vi "GUI_Mlink_Heater.vi"() -> ()   [LabVIEW 2013]
uses:
  Shared/GUI_Template/GUI_master/tcp_new_data_event.ctl
  Shared/GUI_Template/GUI_master/tcp new data cluster.ctl
  <vilib>/Utility/config.llb/Read Key (String).vi
  <vilib>/Utility/config.llb/NI_LVConfig.lvlib
panel:
  in  "Tab Control":enum32{"Plot history", "Configuration", "Debug"}(tab)
  out "Ch1 2":cluster{dbl[], dbl[]}[](graph)
  out "Ch1":cluster{dbl[], dbl[]}[](graph)
  in  "Calibration file path":string="user data\\PL_Energy_meter_callibration.txt"
  in  "Target propagation (%)":dbl=73.68421 format="%_6g"
  in  "Attenuator 2.1 transmittance (%)":dbl format="%_6g"
  in  "Attenuator 2.2 transmittance (%)":dbl=10.1068 format="%_6g"
  in  "Attenuator 1 transmittance (%)":dbl=1.83867 format="%_6g"
  in  "mirror offset (mJ)":dbl
  in  "mirror transmittance (%)":dbl=5.0 format="%_6g"
  out "GUIdevice 1":string="LB-PL-EnergyMeter"
  in  "Select device":string(combo)="LB-PL-EnergyMeter"
  in  "datastream::1":enum16{"off", "on"}(ring)
  in  "polarity::1":enum16{"Positive", "Negative"}(ring) caption="Trigger Polarity"
  out "validdata::1":enum16{"yes", "no"}(ring)
  out "error":errorcluster
  in  "Attenuator 2":enum16{"Out", "In (Att. 2.1)", "In (Att. 2.2)"}(ring)
  in  "Attenuator 1":enum16{"In", "Out"}(ring)=enum."Out"
  in  "Position powermeter":enum16{"In beamline", "Behind mirror"}(ring)=enum."Behind mirror"
  in  "Scale":T1(ring)
  in  "trigger::1":enum16{"Internal", "External"}(ring) caption="Trigger"
  in  "autorange::1":enum16{"off", "on"}(ring) caption="AutoRange"
  out "Target energy (J)":dbl=25.5 min=0.0 max=300000000.0 format="%#_6p"
  out "Full beam energy (J)":dbl=25.5 min=0.0 max=300000000.0 format="%#_6p"
  in  "stop":bool
  in  "data::1":dbl=25.5 caption="Raw energy (J)" min=0.0 max=300000000.0 format="%#_6p"
  in  "Clear 2":bool
  out "tcp data event 2":T2
  in  "insert tag":bool=TRUE
  # "HPD Energy Meter"
  # "Settings"
  # "Aditional settings"
  # "Setup parameters"
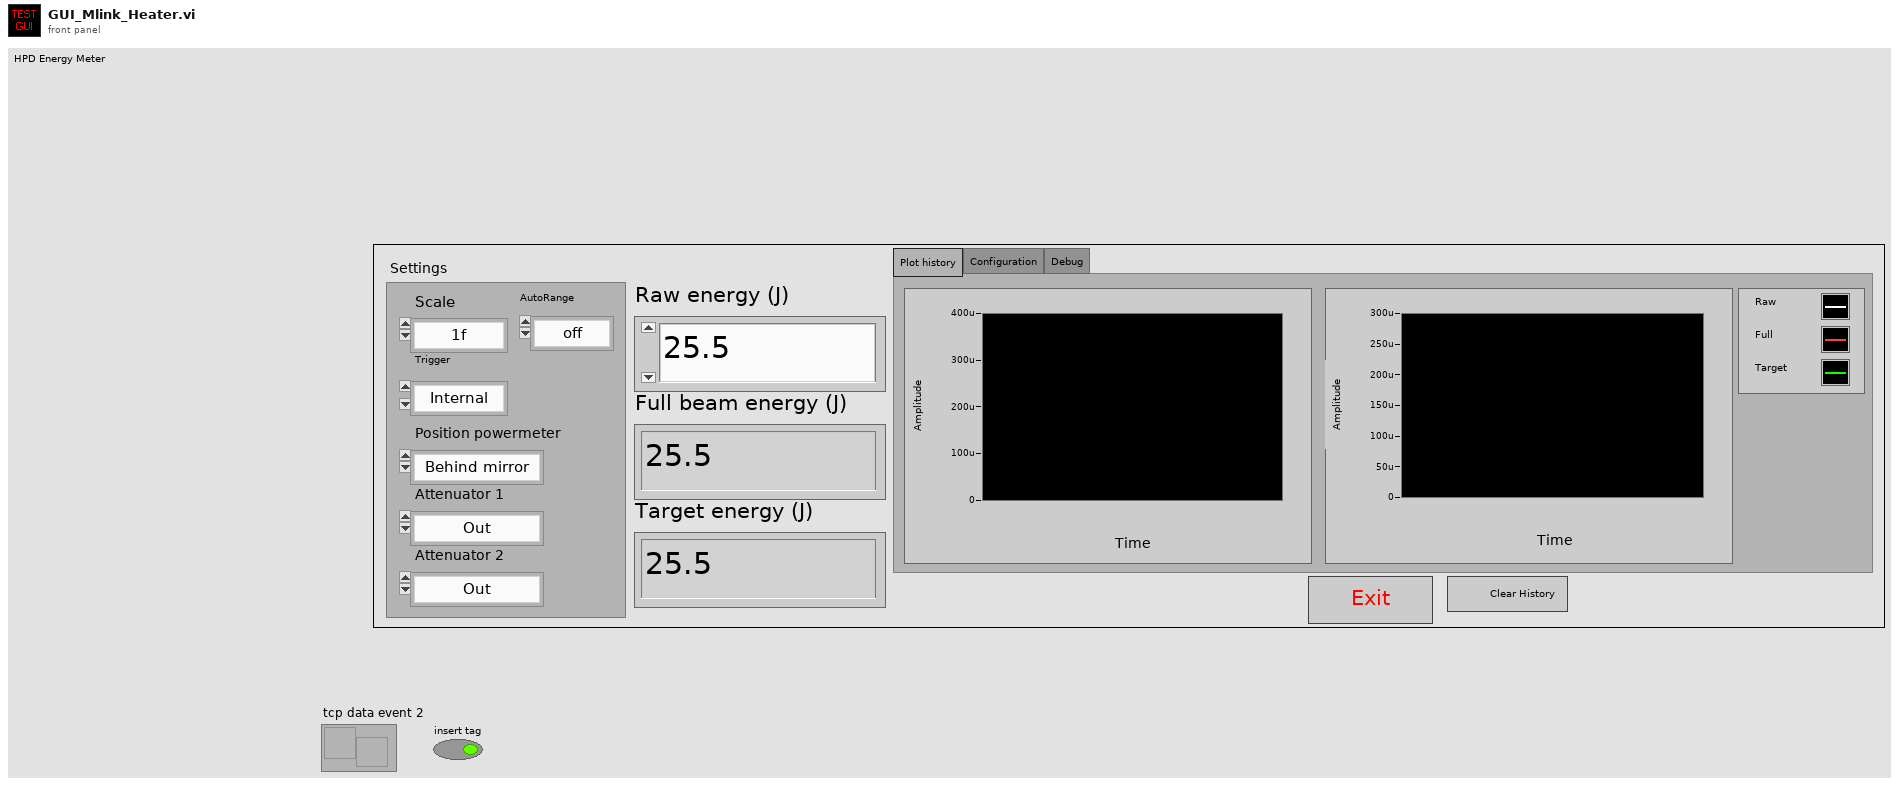
[diagram p1: front panel]
types:
  T1 = enum16{"1f", "3f", "10f", "30f", "100f", "300f", "1p", "3p", "10p", "30p", "100p", "300p", "1n", "3n", "10n", "30n", "100n", "300n", "1u", "3u", "10u", "30u", "100u", "300u", "1m", "3m", "10m", "30m", "100m", "300m", "1", "3", "10", "30", "100", "300", "1K", "3K", "10K", "30K", "100K", "300K", "1M", "3M", "10M", "30M", "100M", "300M"}
  T2 = typedef "tcp_new_data_event.ctl" = refnum<user-event>
  T3 = enum32{"invalid app kind", "Development System", "Run Time System", "Student Edition", "Embedded LabVIEW", "Evaluation", "Custom"}
  T4 = typedef "tcp new data cluster.ctl" = cluster{"EventEnum":enum16{"new data", "connection status update"}, "Device name":string}
  T5 = enum32{"Invalid", "Standard", "Closed", "Hidden", "Minimized", "Maximized"}
  T6 = cluster{"Core":cluster{"Current VI Reference":refnum<vi>, "Close Panel on Exit?":bool}, "Your Boolean data":bool, "Your string data":string, "SuperGUI":cluster{"STOP queue":refnum<queue>, "SuperGUI ref":refnum<vi>, "event reg":refnum<event-registration>}, "Timer":u32, "Raw energy":dbl, "Full energy":dbl, "Target energy":dbl, "Display Error Popup":bool}
  T7 = cluster{"STOP queue":refnum<queue>, "SuperGUI ref":refnum<vi>, "event reg":refnum<event-registration>}
  T8 = cluster{"Current VI Reference":refnum<vi>, "Close Panel on Exit?":bool}
  T9 = typedef "NI_LVConfig.lvlib/Config Data RefNum.ctl" = refnum<k1>
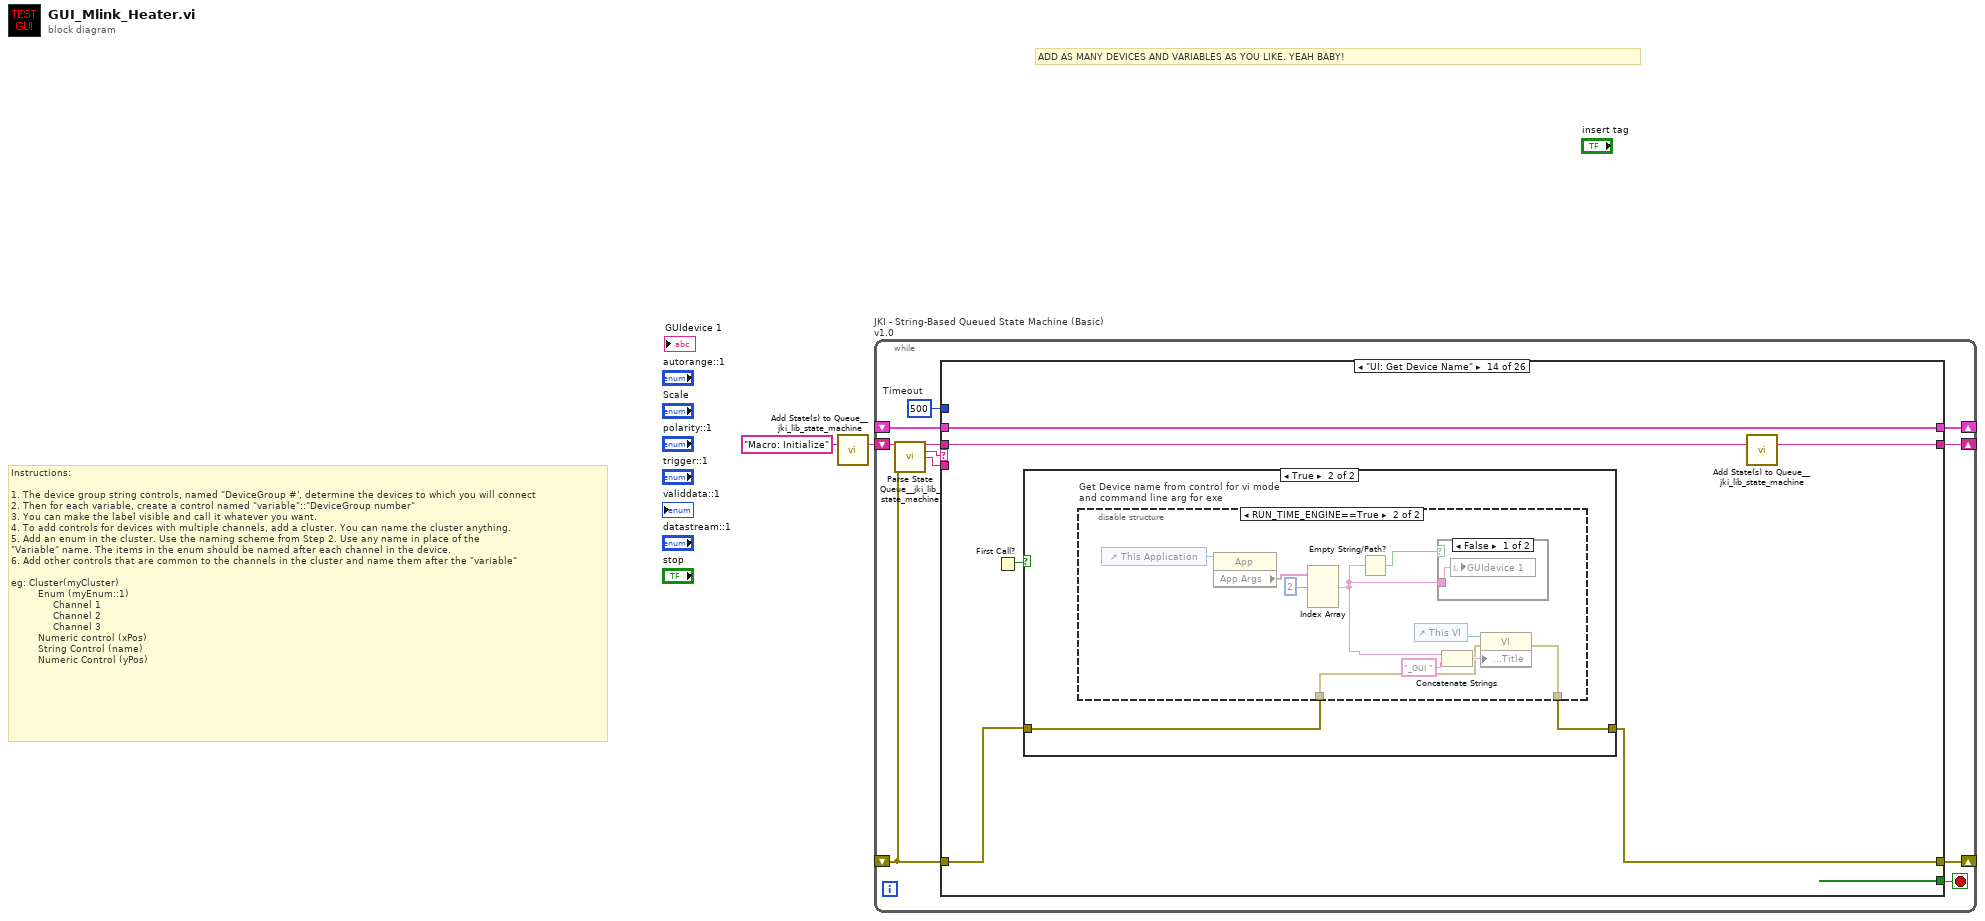
[diagram p0: block diagram]
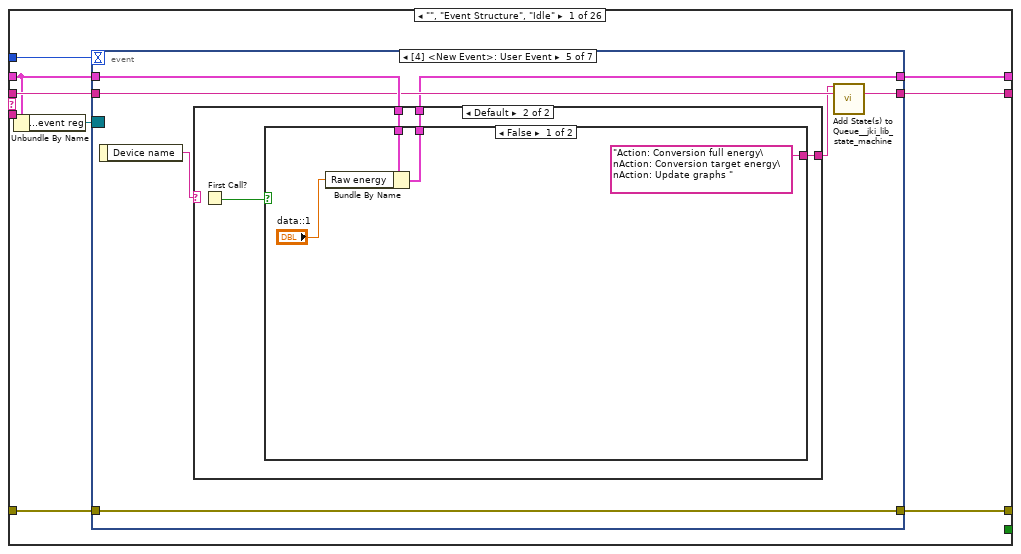
[diagram p2: hidden frame]
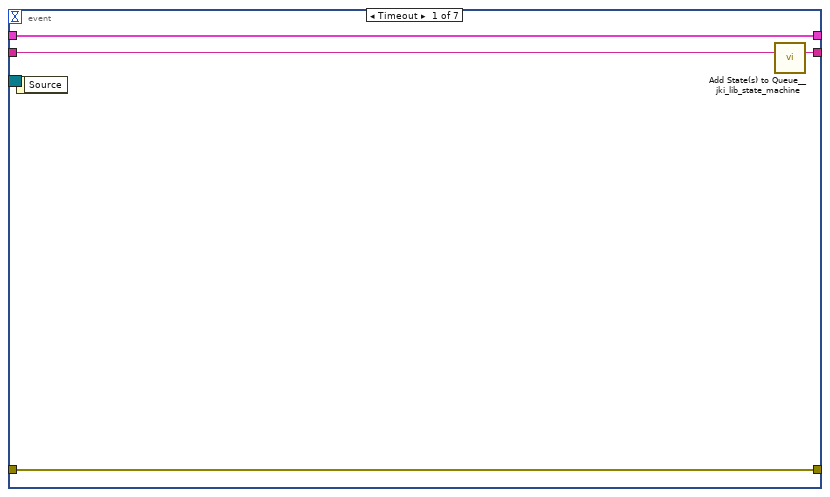
[diagram p3: hidden frame]
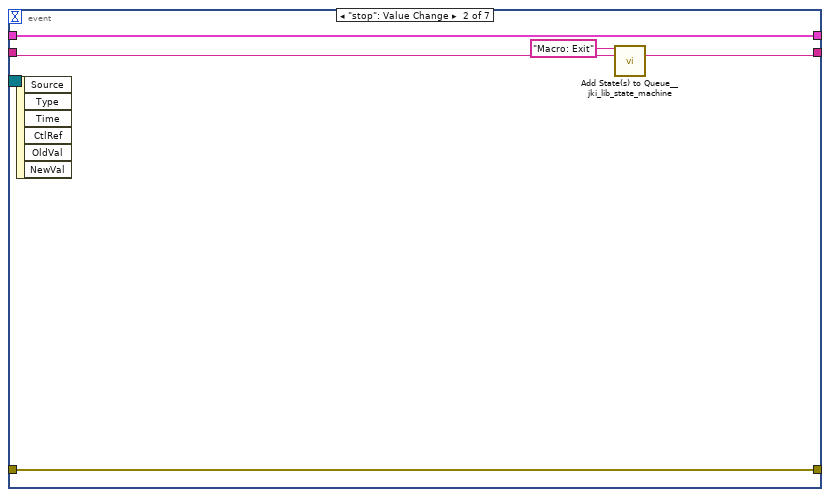
[diagram p4: hidden frame]
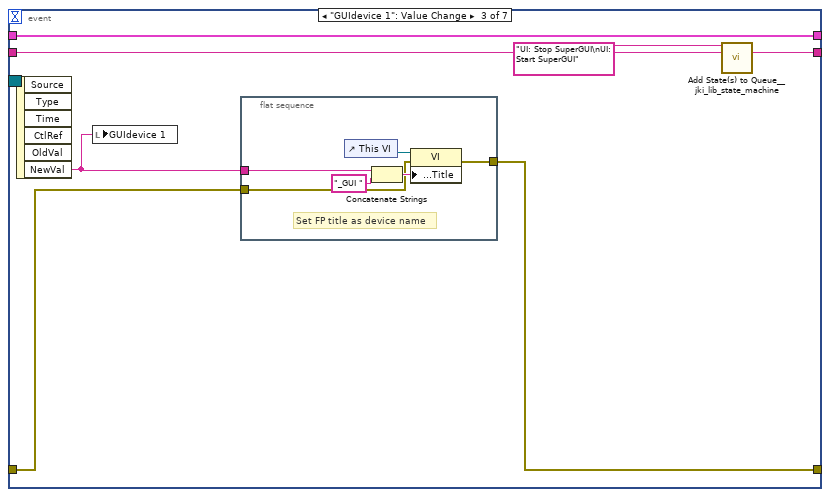
[diagram p5: hidden frame]
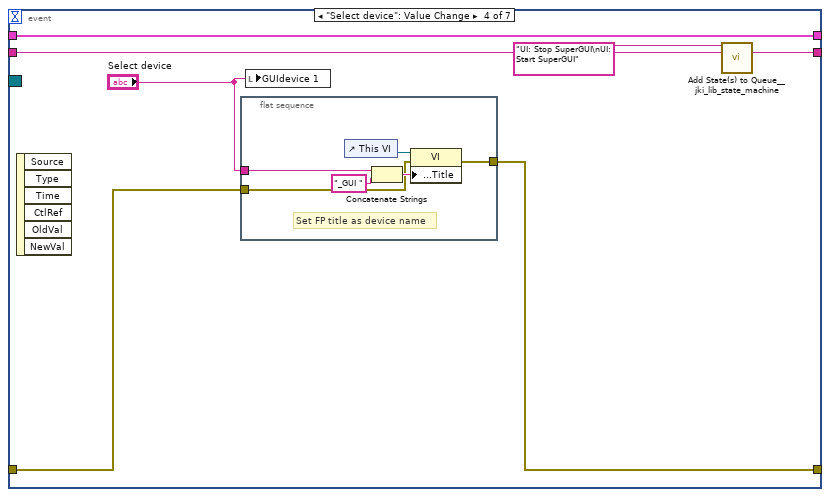
[diagram p6: hidden frame]
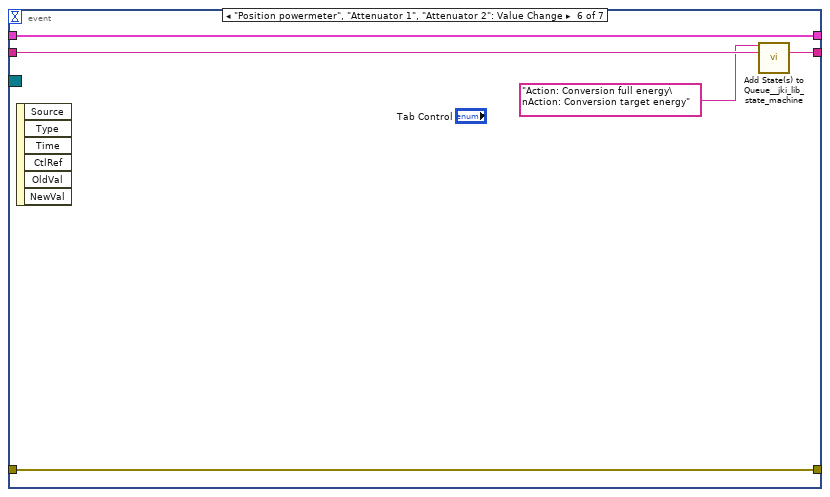
[diagram p9: hidden frame]
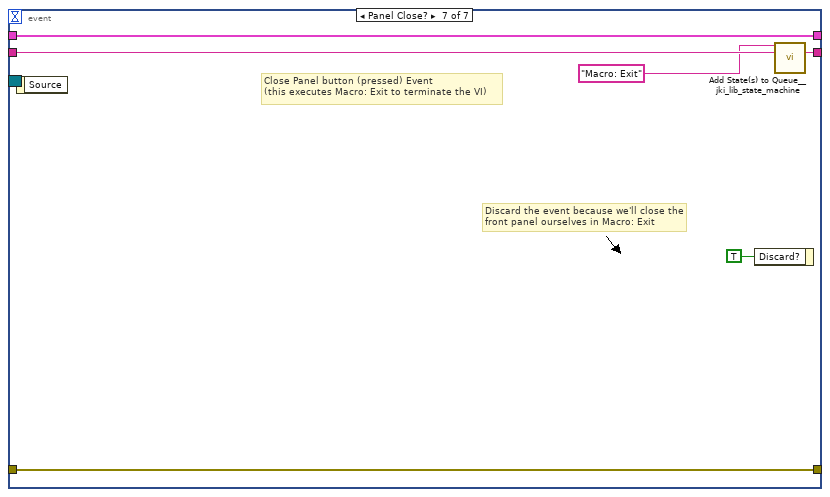
[diagram p10: hidden frame]
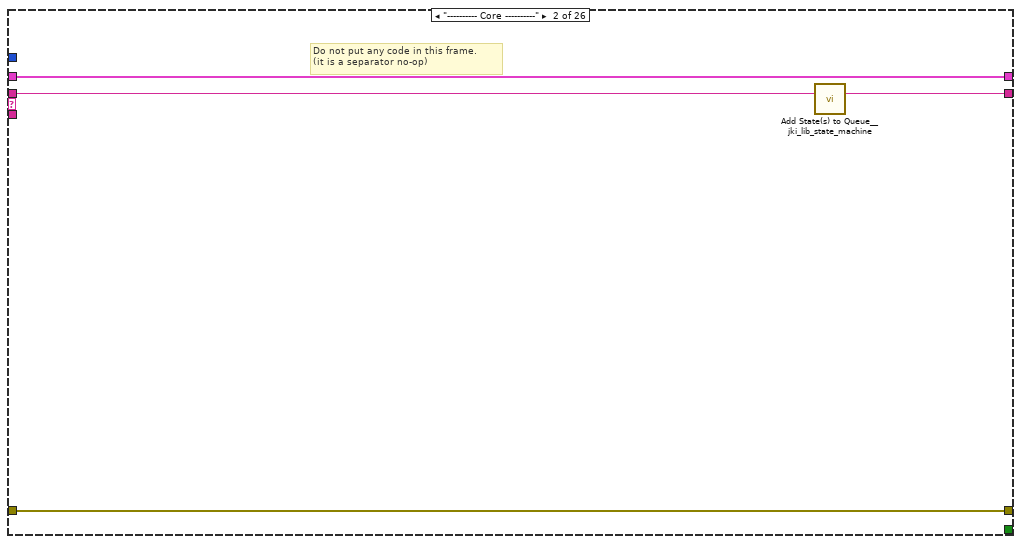
[diagram p11: hidden frame]
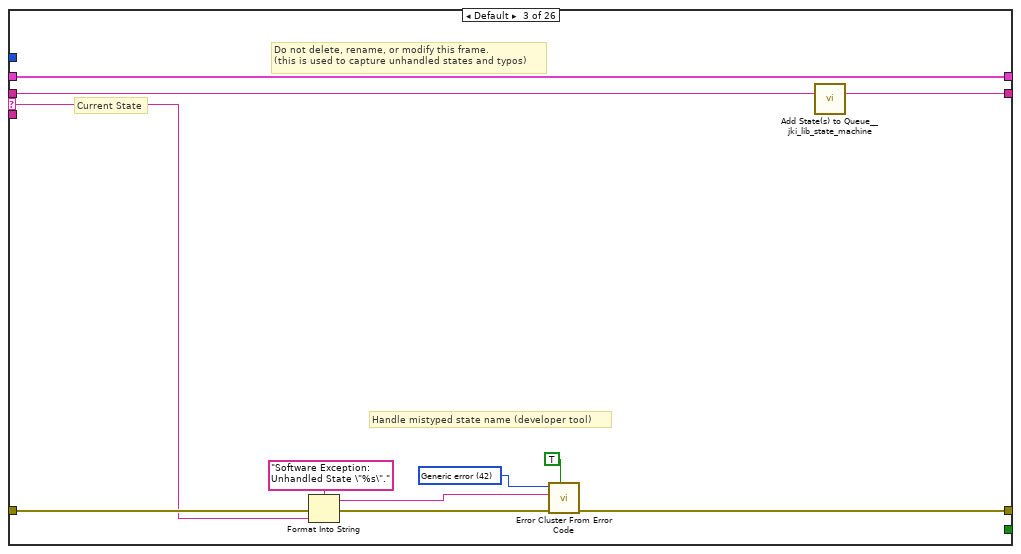
[diagram p12: hidden frame]
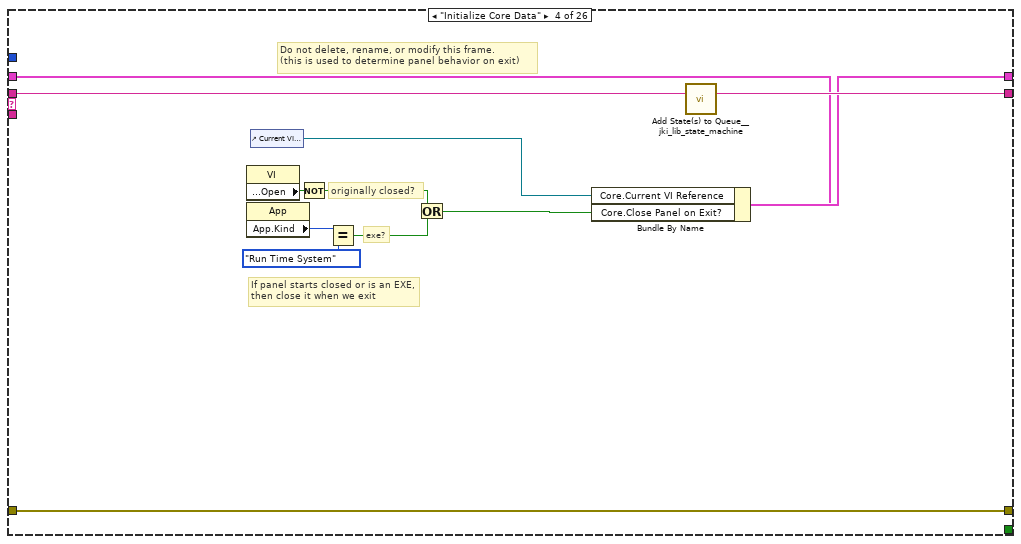
[diagram p13: hidden frame]
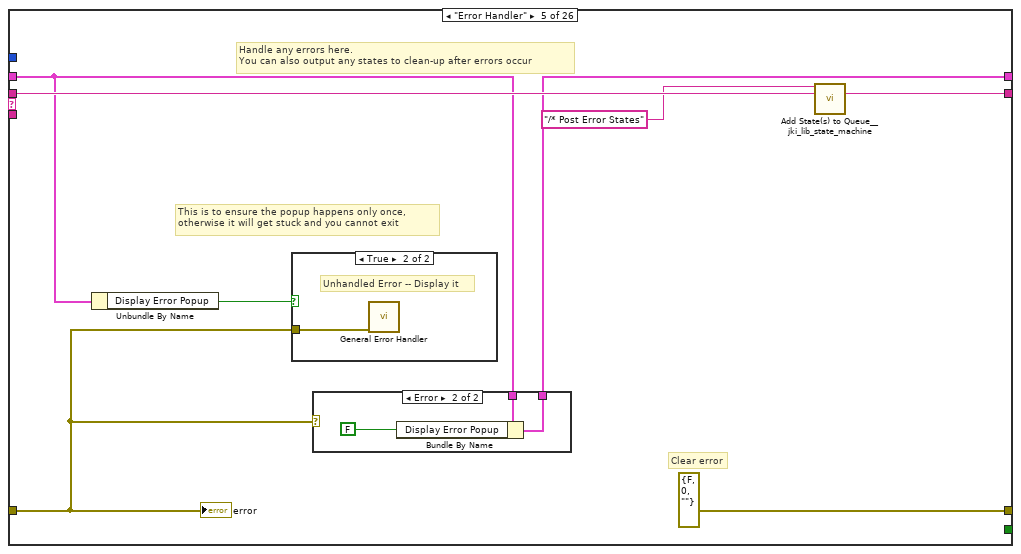
[diagram p14: hidden frame]
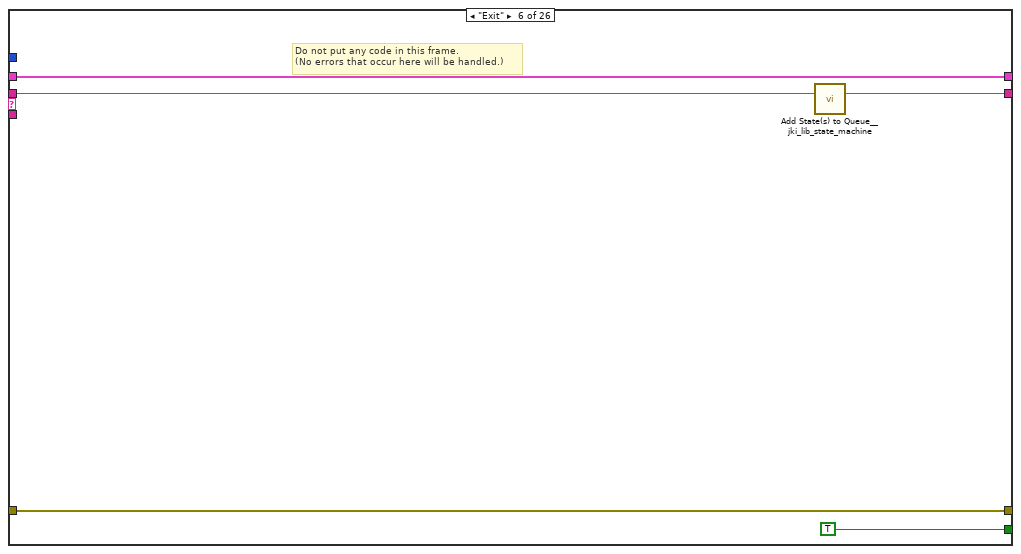
[diagram p17: hidden frame]
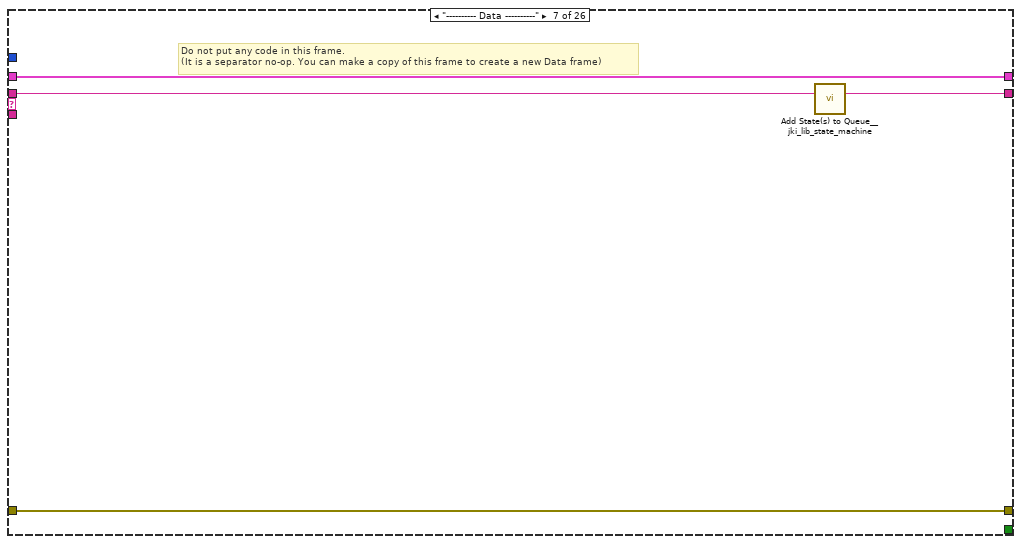
[diagram p18: hidden frame]
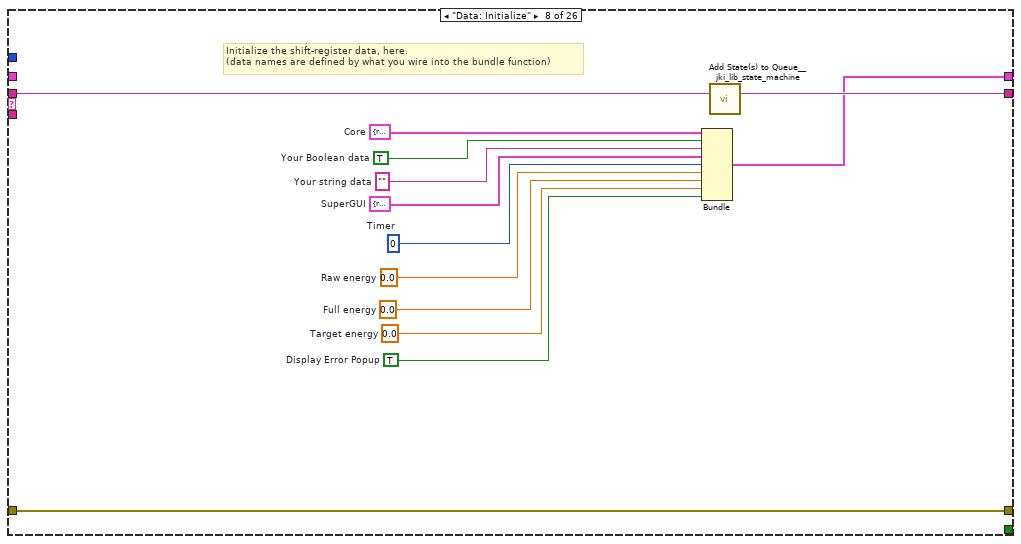
[diagram p19: hidden frame]
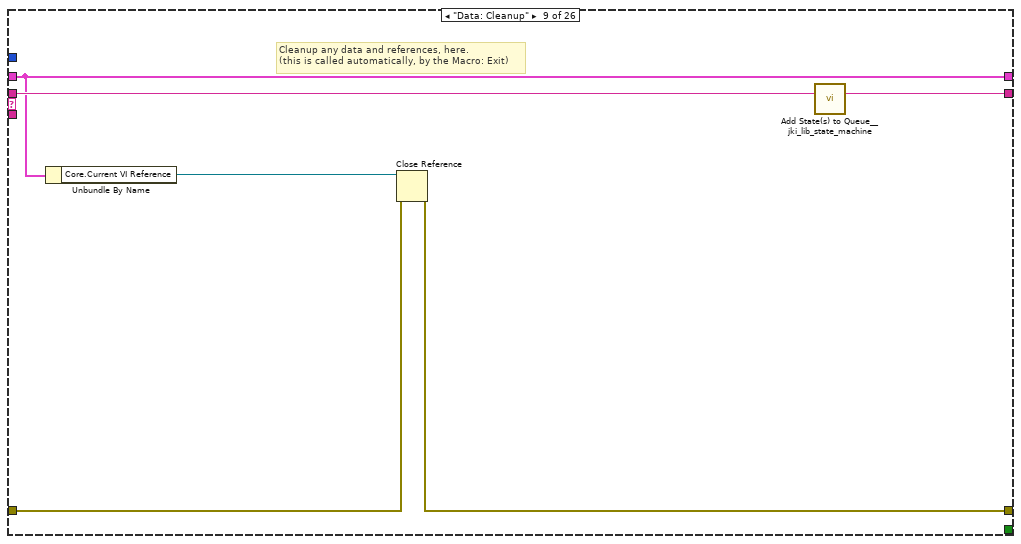
[diagram p20: hidden frame]
diagram:
  # "Instructions:\n\n1. The device group string controls, named \"DeviceGroup #', determine the devices to which you will connect\n2. Then for each variable, create a control named \"variable\"::\"DeviceGroup number\"\n3. You can make the label visible and call it whatever you want.\n4. To add controls for devices with multiple channels, add a cluster. You can name the cluster anything.\n5. Add an enum in the cluster. Use the naming scheme from Step 2. Use any name in place of the \n\"Variable\" name. The items in the enum should be named after each channel in the device. \n6. Add other controls that are common to the channels in the cluster and name them after the \"variable\"\n\neg: Cluster(myCluster)\n         Enum (myEnum::1)\n              Channel 1 \n              Channel 2\n              Channel 3\n         Numeric control (xPos)\n         String Control (name)\n         Numeric Control (yPos)"
  # "ADD AS MANY DEVICES AND VARIABLES AS YOU LIKE. YEAH BABY!"
  n1 = call <vilib>:"Add State(s) to Queue__jki_lib_state_machine.vi"("State(s) in (\"\")"="Macro: Initialize") -> ("States Out"=w2:string)  [unwired: 14 in]
  n2 = while "JKI - String-Based Queued State Machine (Basic) v1.0" {
    shift-right: [w6] -> _
    shift-left: _ -> [w5]
    shift-right: [w9] -> _
    shift-left: _ -> [w3]
    shift-right: [w8] -> _
    shift-left: w2 -> [w10]
    stop <- w7 stop-if-true
    w4 = 500  # Timeout
    n3 = call <vilib>:"Parse State Queue__jki_lib_state_machine.vi"("State Queue"=w10, "Error In (no error)"=w3) -> ("Remaining States"=w12:string, "Current State"=w13:string, "Arguments"=w11:string)  [unwired: 11 in]
    n4 = case shown="\"UI: Get Device Name\"" w13 {
      selector: w13 -> [_ _ w89 _ _ _ _ _ _ _ _ _ _ _ _ _ _ _ _ _ _ _ _ _ _ _]
      tunnel: w12 -> [w21 w88 w93 w111 w119 w129 w133 w146 w152 w156 w166 w196 w211 w217 w252 w260 w266 w277 w303 w308 w318 w322 w330 w351 w386 w412]
      tunnel: w11 -> [_ _ _ _ _ _ _ _ _ _ _ _ _ _ _ _ w261 w271 _ _ _ _ _ _ _ _]
      tunnel: w5 -> [w15 w85 w91 w102 w113 w127 w130 _ w147 w153 w159 w197 w209 w215 w243 w255 w264 w273 w300 w305 w315 w319 w327 w350 w379 w409]
      tunnel: [w19 w86 w95 w108 errorcluster {"status"=FALSE, "code"=0, "source"=""} ("error out") w126 w131 w143 w148 w154 w163 w182 w208 w212 w236 w253 w262 w274 w301 w306 w316 w320 w328 w353 w384 w410] -> w9
      tunnel: w3 -> [w18 w86 w94 w108 w114 w126 w131 w143 w149 w154 w164 w186 w208 w213 w237 w254 w263 w275 w301 w306 w316 w320 w328 w353 w384 w410]
      tunnel: [w20 w87 w92 w110 w118 w128 w132 w145 w151 w155 w165 w196 w210 w216 w251 w259 w265 w276 w302 w307 w317 w321 w329 w354 w385 w411] -> w8
      tunnel: [_ _ _ _ _ TRUE _ _ _ _ _ _ _ _ _ _ _ _ _ _ _ _ _ _ _ _] -> w7
      tunnel: [w17 w85 w91 w109 w112 w127 w130 w144 w147 w153 w158 w197 w209 w215 w242 w255 w264 w273 w300 w305 w315 w319 w326 w349 w380 w409] -> w6
      tunnel: w4 -> [w16 _ _ _ _ _ _ _ _ _ _ _ _ _ _ _ _ _ _ _ _ _ _ _ _ _]
      frame "", "Event Structure", "Idle" {
        n5 = Unbundle By Name(w15) -> ("SuperGUI.event reg"=w14:refnum<event-registration>)
        n6 = event shown="[4] <New Event>: User Event" {
          selector: w14 -> [_ _ _ _ _ _ _]
          dyn-events: _ -> [_ _ _ _ _ _ _]
          timeout: w16 -> [_ _ _ _ _ _ _]
          tunnel: w21 -> [w25 w28 w34 w47 w59 w75 w84]
          tunnel: [w24 w27 w33 w46 w60 w76 w83] -> w20
          tunnel: w15 -> [w22 w30 w37 w50 w61 w77 w81]
          tunnel: [w23 w29 w35 w48 w63 w78 w82] -> w19
          tunnel: w18 -> [w23 w29 w36 w49 w63 w78 w82]
          tunnel: [w22 w30 w37 w50 w57 w77 w81] -> w17
          event Timeout {
            n7 = event-data() -> ()  [unwired: 1 in, 1 out]
            n8 = call <vilib>:"Add State(s) to Queue__jki_lib_state_machine.vi"("State(s) in (\"\")"=w25) -> ("States Out"=w24:string)  [unwired: 14 in]
          }
          event "stop": Value Change {
            n9 = event-data() -> ()  [unwired: 1 in, 6 out]
            n10 = call <vilib>:"Add State(s) to Queue__jki_lib_state_machine.vi"("State(s) in Front (\"\")"="Macro: Exit", "State(s) in (\"\")"=w28) -> ("States Out"=w27:string)  [unwired: 13 in]
          }
          event "GUIdevice 1": Value Change {
            n11 = event-data() -> ("NewVal"=w31:string)  [unwired: 1 in, 5 out]
            n12 = local write "GUIdevice 1"(w31) -> ()
            n13 = flat-sequence {
              tunnel: [w40] -> w35
              tunnel: w36 -> [w39]
              tunnel: w31 -> [w38]
              frame #0 {
                # "Set FP title as device name"
                n14 = control-ref of="This VI"() -> (w43:refnum<vi>)
                n15 = Concatenate Strings(w38, "_GUI ") -> (w42:string)
                n16 = property class="VI"(reference=w43, error in=w39, "Front Panel.Title"=w42) -> (error out=w40:errorcluster)  [unwired: 1 out]
              }
            }
            n17 = call <vilib>:"Add State(s) to Queue__jki_lib_state_machine.vi"("State(s) in Front (\"\")"="UI: Stop SuperGUI\nUI: Start SuperGUI", "State(s) in (\"\")"=w34) -> ("States Out"=w33:string)  [unwired: 13 in]
          }
          event "Select device": Value Change {
            n18 = event-data() -> ()  [unwired: 1 in, 6 out]
            n19 = flat-sequence {
              tunnel: [w53] -> w48
              tunnel: w49 -> [w52]
              tunnel: "Select device" -> [w51]
              frame #0 {
                # "Set FP title as device name"
                n20 = control-ref of="This VI"() -> (w56:refnum<vi>)
                n21 = Concatenate Strings(w51, "_GUI ") -> (w55:string)
                n22 = property class="VI"(reference=w56, error in=w52, "Front Panel.Title"=w55) -> (error out=w53:errorcluster)  [unwired: 1 out]
              }
            }
            n23 = local write "GUIdevice 1"("Select device") -> ()
            n24 = call <vilib>:"Add State(s) to Queue__jki_lib_state_machine.vi"("State(s) in Front (\"\")"="UI: Stop SuperGUI\nUI: Start SuperGUI", "State(s) in (\"\")"=w47) -> ("States Out"=w46:string)  [unwired: 13 in]
          }
          event User Event {
            n25 = event-data() -> ("Device name"=w62:string)  [unwired: 1 in]
            n26 = case shown="Default" w62 {
              tunnel: w61 -> [w64 w67]
              tunnel: [w64 w66] -> w57
              tunnel: [_ w65] -> w58
              frame "" {
              }
              frame Default {
                n27 = First Call?() -> (First Call?: T/F=w68:bool)
                n28 = case shown="False" w68 {
                  tunnel: w67 -> [w72 w73]
                  tunnel: [w71 w73] -> w66
                  tunnel: ["Action: Conversion full energy\nAction: Conversion target energy\nAction: Update graphs " _] -> w65
                  frame False {
                    n29 = Bundle By Name(cluster=w72, "Raw energy"="data::1") -> (w71:T6)
                  }
                  frame True {
                  }
                }
              }
            }
            n30 = call <vilib>:"Add State(s) to Queue__jki_lib_state_machine.vi"("State(s) in Front (\"\")"=w58, "State(s) in (\"\")"=w59) -> ("States Out"=w60:string)  [unwired: 13 in]
          }
          event "Position powermeter", "Attenuator 1", "Attenuator 2": Value Change {
            n31 = event-data() -> ()  [unwired: 1 in, 6 out]
            n32 = call <vilib>:"Add State(s) to Queue__jki_lib_state_machine.vi"("State(s) in Front (\"\")"="Action: Conversion full energy\nAction: Conversion target energy", "State(s) in (\"\")"=w75) -> ("States Out"=w76:string)  [unwired: 13 in]
          }
          event Panel Close? {
            # "Discard the event because we'll close the front panel ourselves in Macro: Exit"
            # "Close Panel button (pressed) Event\n(this executes Macro: Exit to terminate the VI)"
            n33 = event-data() -> ()  [unwired: 1 in, 1 out]
            n34 = event-data("Discard?"=TRUE) -> ()  [unwired: 1 in, 1 out]
            n35 = call <vilib>:"Add State(s) to Queue__jki_lib_state_machine.vi"("State(s) in Front (\"\")"="Macro: Exit", "State(s) in (\"\")"=w84) -> ("States Out"=w83:string)  [unwired: 13 in]
          }
        }
      }
      frame "---------- Core ----------" {
        # "Do not put any code in this frame.\n(it is a separator no-op)"
        n36 = call <vilib>:"Add State(s) to Queue__jki_lib_state_machine.vi"("State(s) in (\"\")"=w88) -> ("States Out"=w87:string)  [unwired: 14 in]
      }
      frame Default {
        w98 = 42 items=["No error", "Argument error", "Memory is full", "Out of zone", "End of file", "File already open", "Generic file I/O error", "File not found", "File permission error", "Disk is full", "Duplicate path", "Too many files open", "System feature not enabled", "Resource file not found", "Cannot add resource", "Resource not found", "Image not found", "Image memory error", "Pen does not exist", "Config type invalid", "Config token not found", "Config parse error", "Config memory error", "Bad external code format", "Bad external code offset", "External code not present", "Null window", "Destroy window error", "Null menu", "Print aborted", "Bad print record", "Print driver error", "Windows error during printing", "Memory error during printing", "Print dialog error", "Generic print error", "Invalid device refnum", "Device not found", "Device parameter error", "Device unit error", "Cannot open device", "Device call aborted", "Generic error", "Cancelled by user", "Object ID too low", "Object ID too high", "Object not in heap", "Unknown heap", "Unknown object (invalid DefProc)", "Unknown object (DefProc not in table)", "Message out of range", "Invalid (null) method", "Unknown message", "Manager call not supported", "Bad address", "Network operation in progress", "Network operation timed out", "Connection is busy", "Network attribute not supported", "Network error", "Address in use", "System out of memory", "Connection aborted", "Connection refused", "Not connected", "Already connected", "Connection closed", "Initialization error (interapplication manager)", "Bad occurrence", "Wait on unbound occurrence handler", "Occurrence queue overflow", "Datalog type conflict", "Unused", "Unrecognized type (interapplication manager)", "Memory corrupt", "Failed to make temporary DLL", "Old CIN version", "Drag socket not found", "Failed to load drop-object", "Failed to register OLE object", "Failed to release OLE object", "Format specifier type mismatch", "Unknown format specifier", "Too few format specifiers", "Too many format specifiers", "Scan failed", "Newer CIN version", "Error converting to variant", "Runtime menu error", "Password tampered", "Variant attribute not found", "Incompatible variant data type", "Event data is not available", "Event Store is not present", "Occurrence is not found", "Event Queue is not created", "Event info is not available", "Refnum passed is NULL", "Error retrieving Class GUID", "Error retrieving CoClass GUID", "Error retrieving TypeLib GUID.", "Bad built application magic bytes.", "Specific driver is different from the specific driver associated with the Logical Name.", "There is no session opened to the class driver.", "Max Error", "MAX - Error with config objects", "MAX - Error loading configuration", "MAX - Group not supported"]
        # "Current State"
        # "Do not delete, rename, or modify this frame.\n(this is used to capture unhandled states and typos)"
        # "Handle mistyped state name (developer tool)"
        n37 = Format Into String(format string="Software Exception: Unhandled State \"%s\"." ("message"), error in=w94, w89) -> (resulting string=w97:string, error out=w96:errorcluster)  [unwired: 1 in]
        n38 = call <vilib>:"Error Cluster From Error Code.vi"("show call chain? (False)"=TRUE, "error in (no error)"=w96, "error message (\"\")"=w97, "error code (0)"=w98) -> ("error out"=w95:errorcluster)  [unwired: 5 in]
        n39 = call <vilib>:"Add State(s) to Queue__jki_lib_state_machine.vi"("State(s) in (\"\")"=w93) -> ("States Out"=w92:string)  [unwired: 14 in]
      }
      frame "Initialize Core Data" {
        # "Do not delete, rename, or modify this frame.\n(this is used to determine panel behavior on exit)"
        # "originally closed?"
        # "exe?"
        # "If panel starts closed or is an EXE, then close it when we exit"
        n40 = property class="VI"() -> ("Front Panel.Open"=w107:bool)  [unwired: 2 in, 2 out]
        n41 = property class="App"() -> ("App.Kind"=w106:T3)  [unwired: 2 in, 2 out]
        n42 = control-ref of="Current VI Reference"() -> (w100:refnum<vi>)
        n43 = Not(x=w107) -> (.not. x?=w104:bool)
        n44 = Equal?(x=w106, y=T3."Run Time System" ("Application:Kind")) -> (x = y?=w103:bool)
        n45 = Or(x=w104, y=w103) -> (x .or. y?=w101:bool)
        n46 = Bundle By Name(cluster=w102, "Core.Current VI Reference"=w100, "Core.Close Panel on Exit?"=w101) -> (w109:T6)
        n47 = call <vilib>:"Add State(s) to Queue__jki_lib_state_machine.vi"("State(s) in (\"\")"=w111) -> ("States Out"=w110:string)  [unwired: 14 in]
      }
      frame "Error Handler" {
        # "This is to ensure the popup happens only once, \notherwise it will get stuck and you cannot exit"
        # "Handle any errors here.\nYou can also output any states to clean-up after errors occur"
        # "Clear error"
        n48 = Unbundle By Name(w113) -> ("Display Error Popup"=w115:bool)
        n49 = case shown="True" w115 {
          tunnel: w114 -> [_ w120]
          frame False {
          }
          frame True {
            # "Unhandled Error -- Display it"
            n50 = call <vilib>:"General Error Handler.vi"("error in (no error)"=w120) -> ()  [unwired: 10 in, 5 out]
          }
        }
        n51 = case shown="Error" w114 {
          tunnel: w113 -> [w121 w124]
          tunnel: [w121 w123] -> w112
          frame No Error {
          }
          frame Error {
            n52 = Bundle By Name(cluster=w124, "Display Error Popup"=FALSE) -> (w123:T6)
          }
        }
        n53 = call <vilib>:"Add State(s) to Queue__jki_lib_state_machine.vi"("State(s) in Front (\"\")"="/* Post Error States", "State(s) in (\"\")"=w119) -> ("States Out"=w118:string)  [unwired: 13 in]
        "error" <- w114
      }
      frame "Exit" {
        # "Do not put any code in this frame.\n(No errors that occur here will be handled.)"
        n54 = call <vilib>:"Add State(s) to Queue__jki_lib_state_machine.vi"("State(s) in (\"\")"=w129) -> ("States Out"=w128:string)  [unwired: 14 in]
      }
      frame "---------- Data ----------" {
        # "Do not put any code in this frame.\n(It is a separator no-op. You can make a copy of this frame to create a new Data frame)"
        n55 = call <vilib>:"Add State(s) to Queue__jki_lib_state_machine.vi"("State(s) in (\"\")"=w133) -> ("States Out"=w132:string)  [unwired: 14 in]
      }
      frame "Data: Initialize" {
        w134 = TRUE  # Display Error Popup
        w135 = 0.0  # Target energy
        w136 = 0.0  # Full energy
        w137 = 0.0  # Raw energy
        w138 = u32 0  # Timer
        w139 = T7 {"STOP queue"=refnum, "SuperGUI ref"=refnum, "event reg"=refnum}  # SuperGUI
        w140 = T8 {"Current VI Reference"=refnum, "Close Panel on Exit?"=FALSE}  # Core
        w142 = TRUE  # Your Boolean data
        w141 = ""  # Your string data
        # "Initialize the shift-register data, here.\n(data names are defined by what you wire into the bundle function)"
        n56 = Bundle("Core"=w140, "Your Boolean data"=w142, "Your string data"=w141, "SuperGUI"=w139, "Timer"=w138, "Raw energy"=w137, "Full energy"=w136, "Target energy"=w135, "Display Error Popup"=w134) -> (w144:T6)  [unwired: 1 in]
        n57 = call <vilib>:"Add State(s) to Queue__jki_lib_state_machine.vi"("State(s) in (\"\")"=w146) -> ("States Out"=w145:string)  [unwired: 14 in]
      }
      frame "Data: Cleanup" {
        # "Cleanup any data and references, here.\n(this is called automatically, by the Macro: Exit)"
        n58 = Unbundle By Name(w147) -> ("Core.Current VI Reference"=w150:refnum<vi>)
        n59 = Close Reference(reference=w150, error in (no error)=w149) -> (error out=w148:errorcluster)
        n60 = call <vilib>:"Add State(s) to Queue__jki_lib_state_machine.vi"("State(s) in (\"\")"=w152) -> ("States Out"=w151:string)  [unwired: 14 in]
      }
      frame "---------- UI ----------" {
        # "Do not put any code in this frame.\n(It is a separator no-op. You can make a copy of this frame to create a new UI frame)"
        n61 = call <vilib>:"Add State(s) to Queue__jki_lib_state_machine.vi"("State(s) in (\"\")"=w156) -> ("States Out"=w155:string)  [unwired: 14 in]
      }
      frame "UI: Initialize" {
        # "Initialize the User Interface, here.\n(this is called automatically, by the Macro: Init)"
        n62 = local read "GUIdevice 1"() -> (w160:string)
        n63 = call <userlib>:"Fit VI window to Largest Dec__ogtk.vi"("error in (no error)"=w164) -> ("error out"=w163:errorcluster)  [unwired: 5 in, 1 out]
        n64 = call "getDevices.vi"("Device Class"="Gentec Mlink") -> ("All Devices"=w162:string[])
        n65 = property on="Select device" class="CmbBox"("Strings[]"=w162, "Value"=w160) -> ()  [unwired: 2 in, 2 out]
        n66 = call <userlib>:"Tick Count (ms)__ogtk.vi"() -> ("millisecond timer value"=w157:u32)  [unwired: 10 in, 1 out]
        n67 = Bundle By Name(cluster=w159, "Timer"=w157) -> (w158:T6)
        n68 = call <vilib>:"Add State(s) to Queue__jki_lib_state_machine.vi"("State(s) in (\"\")"=w166) -> ("States Out"=w165:string)  [unwired: 14 in]
      }
      frame "UI: Read callibration txt" {
        n69 = call "get software root directory.vi"() -> ("Application Directory"=w193:path)  [unwired: 11 in]
        n70 = Strip Path(path=w193) -> (stripped path=w192:path)  [unwired: 1 out]
        n71 = Build Path(base path=w192, name or relative path="Calibration file path") -> (appended path=w191:path)
        n72 = call <vilib>:"Open Config Data.vi"("error in (no error)"=w186, "create file if necessary (T)"=FALSE, "configuration file path"=w191) -> ("error out"=w190:errorcluster, "refnum"=w189:T9)  [unwired: 6 in, 1 out]
        n73 = for {
          tunnel: [w207] -> w185 mode=indexing
          tunnel: w189 -> [w204]
          tunnel: string[] ["Target propagation (%)", "mirror transmittance (%)", "mirror offset (mJ)", "Attenuator 1 transmittance (%)", "Attenuator 2.1 transmittance (%)", "Attenuator 2.2 transmittance (%)"] -> [w203] mode=indexing
          tunnel: "LB-PL-EnergyMeter" ("key") -> [w202]
          tunnel: [w200] -> w181 mode=indexing
          shift-right: [w206] -> w173
          shift-left: w190 -> [w205]
          n74 = call-poly <vilib>:"Read Key.vi"("section"=w202, "error in (no error)"=w205, "default value"="", "key"=w203, "refnum"=w204) -> ("error out"=w206:errorcluster, "value"=w200:string, "found?"=w207:bool)  [unwired: 3 in, 1 out]
        }
        n75 = Fract/Exp String To Number(string=w181) -> (number=w180:dbl[])  [unwired: 3 in, 1 out]
        n76 = And Array Elements(Boolean array=w185) -> (logical AND=w183:bool)
        n77 = case shown="False" w183 {
          tunnel: [errorcluster {"status"=TRUE, "code"=0, "source"="[Read from file: Variable not found in .txt file]"} ("error out") errorcluster {"status"=FALSE, "code"=0, "source"=""} ("error out")] -> w184
          frame False {
          }
          frame True {
          }
        }
        n78 = Index Array(array=w180) -> (element #1=w179:dbl, element #2=w178:dbl, element #3=w177:dbl, element #4=w176:dbl, element #5=w175:dbl, element #6=w174:dbl)  [unwired: 6 in]
        n79 = property on="Target propagation (%)" class="DigNum (strict)"(error in=w173, "Val(Sgnl)"=w179) -> (error out=w172:errorcluster)  [unwired: 1 in, 1 out]
        n80 = property on="mirror transmittance (%)" class="DigNum (strict)"(error in=w172, "Val(Sgnl)"=w178) -> (error out=w171:errorcluster)  [unwired: 1 in, 1 out]
        n81 = property on="mirror offset (mJ)" class="DigNum (strict)"(error in=w171, "Val(Sgnl)"=w177) -> (error out=w170:errorcluster)  [unwired: 1 in, 1 out]
        n82 = property on="Attenuator 1 transmittance (%)" class="DigNum (strict)"(error in=w170, "Val(Sgnl)"=w176) -> (error out=w169:errorcluster)  [unwired: 1 in, 1 out]
        n83 = property on="Attenuator 2.1 transmittance (%)" class="DigNum (strict)"(error in=w169, "Val(Sgnl)"=w175) -> (error out=w168:errorcluster)  [unwired: 1 in, 1 out]
        n84 = property on="Attenuator 2.2 transmittance (%)" class="DigNum (strict)"(error in=w168, "Val(Sgnl)"=w174) -> (error out=w167:errorcluster)  [unwired: 1 in, 1 out]
        n85 = Merge Errors(w167, w184) -> (w182:errorcluster)
      }
      frame "UI: Update Device List" {
        n86 = call <vilib>:"Add State(s) to Queue__jki_lib_state_machine.vi"("State(s) in (\"\")"=w211) -> ("States Out"=w210:string)  [unwired: 14 in]
      }
      frame "UI: Get Device Name" {
        n87 = First Call?() -> (First Call?: T/F=w214:bool)
        n88 = case shown="True" w214 {
          tunnel: w213 -> [w218 w220]
          tunnel: [w218 w219] -> w212
          frame False {
          }
          frame True {
            n89 = disable-structure "Get Device name from control for vi mode\nand command line arg for exe" shown="RUN_TIME_ENGINE==True" {
              disable-tunnel: w220 -> [_ w222]
              disable-tunnel: [_ w221] -> w219
              frame condition #0 (active) {
              }
              frame condition #1 {
                n90 = control-ref of="This Application"() -> (w230:refnum<vi>)
                n91 = property class="App"(reference=w230) -> ("App.Args"=w229:string[])  [unwired: 1 in, 2 out]
                n92 = Index Array(array=w229, index #1=2 ("index")) -> (element #1=w223:string)  [unwired: 2 in, 2 out]
                n93 = Empty String/Path?(string/path=w223) -> (empty?=w227:bool)
                n94 = control-ref of="This VI"() -> (w226:refnum<vi>)
                n95 = case shown="False" w227 {
                  tunnel: w223 -> [w231 _]
                  frame False {
                    n96 = local write "GUIdevice 1"(w231) -> ()
                  }
                  frame True {
                  }
                }
                n97 = Concatenate Strings(w223, "_GUI ") -> (w225:string)
                n98 = property class="VI"(reference=w226, error in=w222, "Front Panel.Title"=w225) -> (error out=w221:errorcluster)  [unwired: 1 out]
              }
            }
          }
        }
        n99 = call <vilib>:"Add State(s) to Queue__jki_lib_state_machine.vi"("State(s) in (\"\")"=w217) -> ("States Out"=w216:string)  [unwired: 14 in]
      }
      frame "UI: Start SuperGUI" {
        # "create stop queue for supergui and its clones"
        # "x100 abort will be dependent on caller VI\nx80 abort will be independent of caller vi, this will abort vi when labview is closed."
        # "Start SuperGUI asynchronous way"
        n100 = vi-ref "GUI_Master_subvi_reentrant_queues.vi"() -> (w235:refnum<vi>)
        n101 = property class="VI"(reference=w235) -> ("Path"=w234:path)  [unwired: 1 in, 2 out]
        n102 = Create User Event(user event datatype=T4 {"EventEnum"=enum."new data", "Device name"="Device name"} ("New Event"), error in=w237) -> (user event=w238:refnum<user-event>, error out=w244:errorcluster)
        "tcp data event 2" <- w238
        n103 = control-ref of="This Application"() -> (w241:refnum<vi>)
        n104 = control-ref of="This VI"() -> (w240:refnum<vi>)
        n105 = Open VI Reference(type specifier VI Refnum (for type only)=refnum<vi> refnum, vi path=w234, options=256) -> (vi reference=w250:refnum<vi>, error out=w249:errorcluster)  [unwired: 3 in]
        n106 = register-events(w238) -> (reference out=w232:refnum<event-registration>)  [unwired: 2 in, 1 out]
        n107 = call "supergui create stop queue.vi"() -> ("STOP Queue out"=w246:refnum<queue>)  [unwired: 11 in]
        n108 = Current VI's Menubar() -> (w239:refnum<k9>)
        n109 = call-by-ref "Start Asynchronous Call"(reference=w250, error in=w249, "STOP Queue in"=w246, "This Application"=w241, 8:"error in (no error)"=w244, "tcp data event"=w238, "Caller menu reference"=w239, "Caller VI ref"=w240) -> (reference out=w233:refnum<vi>, error out=w236:errorcluster)  [unwired: 5 in, 1 out]
        n110 = Bundle By Name(cluster=w243, "SuperGUI.event reg"=w232, "SuperGUI.SuperGUI ref"=w233, "SuperGUI.STOP queue"=w246) -> (w242:T6)
        n111 = call <vilib>:"Add State(s) to Queue__jki_lib_state_machine.vi"("State(s) in (\"\")"=w252) -> ("States Out"=w251:string)  [unwired: 14 in]
      }
      frame "UI: Stop SuperGUI" {
        # "Stop Supergui Clone and wait until it exit properly"
        n112 = Unbundle By Name(w255) -> ("SuperGUI.SuperGUI ref"=w257:refnum<vi>, "SuperGUI.STOP queue"=w256:refnum<queue>)
        n113 = Release Queue(queue=w256, error in (no error)=w254) -> (error out=w258:errorcluster)  [unwired: 1 in, 2 out]
        n114 = call-by-ref "Wait On Asynchronous Call"(reference=w257, error in=w258) -> ("error out"=w253:errorcluster)  [unwired: 11 in, 2 out]
        n115 = call <vilib>:"Add State(s) to Queue__jki_lib_state_machine.vi"("State(s) in (\"\")"=w260) -> ("States Out"=w259:string)  [unwired: 14 in]
      }
      frame "UI: Cursor Set" {
        # "Argument"
        # "Set and Unset Cursor Busy.\n(Usage: \"UI: Cursor Set >> Busy|Idle\")"
        n116 = case shown="\"Idle\", Default" w261 {
          tunnel: w263 -> [w268 w270]
          tunnel: [w267 w269] -> w262
          frame "Idle", Default {
            n117 = call <vilib>:"Unset Busy.vi"("error in (no error)"=w268) -> ("error out"=w267:errorcluster)  [unwired: 10 in]
          }
          frame "Busy" {
            n118 = call <vilib>:"Set Busy.vi"("error in (no error)"=w270) -> ("error out"=w269:errorcluster)  [unwired: 9 in, 1 out]
          }
        }
        n119 = call <vilib>:"Add State(s) to Queue__jki_lib_state_machine.vi"("State(s) in (\"\")"=w266) -> ("States Out"=w265:string)  [unwired: 14 in]
      }
      frame "UI: Front Panel State" {
        # "Argument"
        # "Set Front Panel Open or Closed\n(Usage: \"UI: Front Panel State >> Open|Close\")"
        n120 = Unbundle By Name(w273) -> ("Core.Current VI Reference"=w272:refnum<vi>)
        n121 = case shown="\"Open\", Default" w271 {
          tunnel: w275 -> [w281 w294]
          tunnel: [w283 w295] -> w274
          tunnel: w272 -> [w282 w292]
          frame "Open", Default {
            n122 = property class="VI"(reference=w282, error in=w281) -> (reference out=w279:refnum<vi>, error out=w280:errorcluster, "Front Panel.Open"=w278:bool)
            n123 = case shown="False" w278 {
              tunnel: [w286 w289] -> w283
              tunnel: w280 -> [w285 w289]
              tunnel: w279 -> [w284 _]
              frame False {
                n124 = invoke class="VI" method="FP.Open"(reference=w284, error in=w285, "Activate"=TRUE, "State"=T5."Standard") -> (error out=w286:errorcluster)  [unwired: 1 in, 4 out]
              }
              frame True {
              }
            }
          }
          frame "Close" {
            n125 = property class="VI"(reference=w292, error in=w294) -> (reference out=w291:refnum<vi>, error out=w293:errorcluster, "Front Panel.Open"=w290:bool)
            n126 = case shown="True" w290 {
              tunnel: [w296 w299] -> w295
              tunnel: w293 -> [w296 w298]
              tunnel: w291 -> [_ w297]
              frame False {
              }
              frame True {
                n127 = invoke class="VI" method="FP.Close"(reference=w297, error in=w298) -> (error out=w299:errorcluster)  [unwired: 1 in, 2 out]
              }
            }
          }
        }
        n128 = call <vilib>:"Add State(s) to Queue__jki_lib_state_machine.vi"("State(s) in (\"\")"=w277) -> ("States Out"=w276:string)  [unwired: 14 in]
      }
      frame "---------- Macro ----------" {
        # "Do not put any code in this frame.\n(It is a separator no-op. You can make a copy of this frame to create a new Macro frame)"
        n129 = call <vilib>:"Add State(s) to Queue__jki_lib_state_machine.vi"("State(s) in (\"\")"=w303) -> ("States Out"=w302:string)  [unwired: 14 in]
      }
      frame "Macro: Initialize" {
        # "Initialization Macro\n(This is called once, when the VI starts)"
        n130 = call <vilib>:"Add State(s) to Queue__jki_lib_state_machine.vi"("State(s) in Front (\"\")"="Data: Initialize\nInitialize Core Data\nUI: Initialize\nUI: Read callibration txt\nUI: Update Device List\nUI: Get Device Name\nUI: Start SuperGUI\nUI: Front Panel State >> Open", "State(s) in (\"\")"=w308) -> ("States Out"=w307:string)  [unwired: 13 in]
      }
      frame "Macro: Exit" {
        # "Exit Macro\n(This is called once, when the VI exits)"
        n131 = Unbundle By Name(w315) -> ("Core.Close Panel on Exit?"=w314:bool)
        n132 = Select(t="UI: Front Panel State >> Close", s=w314, f="") -> (s? t:f=w311:string)
        n133 = call <vilib>:"Add State(s) to Queue__jki_lib_state_machine.vi"("State(s) in (\"\")"=w311, "State(s) at Back (\"\")"="Data: Cleanup\nExit") -> ("States Out"=w309:string)  [unwired: 13 in]
        n134 = call <vilib>:"Add State(s) to Queue__jki_lib_state_machine.vi"("State(s) in Front (\"\")"=w309, "State(s) in (\"\")"=w318) -> ("States Out"=w317:string)  [unwired: 13 in]
      }
      frame "---------- Action ----------" {
        # "Template Separator\n(You can make a copy of, or modify, this frame)"
        n135 = call <vilib>:"Add State(s) to Queue__jki_lib_state_machine.vi"("State(s) in (\"\")"=w322) -> ("States Out"=w321:string)  [unwired: 14 in]
      }
      frame "Action: Conversion full energy" {
        n136 = Unbundle By Name(w327) -> ("Raw energy"=w324:dbl)
        n137 = case shown="\"Behind mirror\"" "Position powermeter" {
          tunnel: [w331 w337] -> w323
          tunnel: w324 -> [w331 w338]
          frame "In beamline", Default {
          }
          frame "Behind mirror" {
            n138 = Divide(x="mirror transmittance (%)", y=100.0) -> (x/y=w333:dbl)
            n139 = Reciprocal(x=w333) -> (1/x=w332:dbl)
            n140 = Multiply(x=w338, y=w332) -> (x*y=w339:dbl)
            n141 = Add(x=w339, y="mirror offset (mJ)") -> (x+y=w337:dbl)
          }
        }
        "Full beam energy (J)" <- w323
        n142 = Bundle By Name(cluster=w327, "Full energy"=w323) -> (w326:T6)
        n143 = call <vilib>:"Add State(s) to Queue__jki_lib_state_machine.vi"("State(s) in (\"\")"=w330) -> ("States Out"=w329:string)  [unwired: 14 in]
      }
      frame "Action: Conversion target energy" {
        n144 = Unbundle By Name(w350) -> ("Full energy"=w348:dbl)
        n145 = case shown="\"In\"" "Attenuator 1" {
          tunnel: w348 -> [w370 w375]
          tunnel: [w370 w372] -> w346
          frame "Out", Default {
          }
          frame "In" {
            n146 = Divide(x="Attenuator 1 transmittance (%)", y=100.0) -> (x/y=w371:dbl)
            n147 = Multiply(x=w375, y=w371) -> (x*y=w372:dbl)
          }
        }
        n148 = case shown="\"In (Att. 2.1)\"" "Attenuator 2" {
          tunnel: [w359 w361 w366] -> w345
          tunnel: w346 -> [w359 w364 w369]
          frame "Out", Default {
          }
          frame "In (Att. 2.1)" {
            n149 = Divide(x="Attenuator 2.1 transmittance (%)", y=100.0) -> (x/y=w360:dbl)
            n150 = Multiply(x=w364, y=w360) -> (x*y=w361:dbl)
          }
          frame "In (Att. 2.2)" {
            n151 = Divide(x="Attenuator 2.2 transmittance (%)", y=100.0) -> (x/y=w365:dbl)
            n152 = Multiply(x=w369, y=w365) -> (x*y=w366:dbl)
          }
        }
        n153 = Divide(x="Target propagation (%)", y=100.0) -> (x/y=w340:dbl)
        n154 = case shown="True" TRUE {
          tunnel: w345 -> [w355 w358]
          tunnel: [w355 w357] -> w344
          tunnel: w340 -> [_ w356]
          frame False {
          }
          frame True {
            n155 = Multiply(x=w358, y=w356) -> (x*y=w357:dbl)
          }
        }
        "Target energy (J)" <- w344
        n156 = Bundle By Name(cluster=w350, "Target energy"=w344) -> (w349:T6)
        n157 = call <vilib>:"Add State(s) to Queue__jki_lib_state_machine.vi"("State(s) in (\"\")"=w351) -> ("States Out"=w354:string)  [unwired: 14 in]
      }
      frame "Action: Update graphs" {
        # "Your code here.\n(You can make a copy of, or modify, this frame)"
        n158 = Unbundle By Name(w379) -> ("Raw energy"=w378:dbl, "Full energy"=w376:dbl, "Target energy"=w377:dbl)
        n159 = Unbundle By Name(w379) -> ("Timer"=w381:u32)
        n160 = First Call?() -> (First Call?: T/F=w383:bool)
        n161 = case shown="False" w383 {
          tunnel: w381 -> [w394 w408]
          tunnel: [w393 w408] -> w382
          tunnel: w376 -> [w388 _]
          tunnel: w378 -> [w389 _]
          tunnel: w377 -> [w387 _]
          frame False {
            n162 = call <userlib>:"Tick Count (ms)__ogtk.vi"() -> ("millisecond timer value"=w395:u32)  [unwired: 10 in, 1 out]
            n163 = Subtract(x=w395, y=w394) -> (x-y=w397:u32)
            n164 = Greater Or Equal?(x=w397, y=u32 20000 ("min time between updates")) -> (x >= y?=w396:bool)
            n165 = case shown="True" "Clear 2" {
              frame False {
              }
              frame True {
                n166 = local write "Clear 2"(FALSE ("Clear")) -> ()
              }
            }
            n167 = case shown="True" w396 {
              tunnel: w389 -> [_ w402]
              tunnel: [w399 w406] -> w393
              tunnel: w395 -> [_ w406]
              tunnel: w394 -> [w399 _]
              tunnel: "Clear 2" -> [_ w405]
              tunnel: w388 -> [_ w401]
              tunnel: w387 -> [_ w400]
              frame False {
              }
              frame True {
                n168 = call "add values to xy graph 3 plots.vi"("new value 3"=w400, "new value 2"=w401, "new value"=w402, "max # points"=2000 ("max points"), "Clear"=w405) -> ("xy graph"=→"Ch1 2":cluster{dbl[], dbl[]}[])  [unwired: 4 in, 2 out]
              }
            }
            n169 = call "add values to xy graph 3 plots.vi"("new value 3"=w387, "new value 2"=w388, "new value"=w389, "max # points"=500 ("max points"), "Clear"="Clear 2") -> ("xy graph"=→"Ch1":cluster{dbl[], dbl[]}[])  [unwired: 4 in, 2 out]
          }
          frame True {
          }
        }
        n170 = Bundle By Name(cluster=w379, "Timer"=w382) -> (w380:T6)
        n171 = call <vilib>:"Add State(s) to Queue__jki_lib_state_machine.vi"("State(s) in (\"\")"=w386) -> ("States Out"=w385:string)  [unwired: 14 in]
      }
      frame "Copy me" {
        # "Your code here.\n(You can make a copy of, or modify, this frame)"
        n172 = call <vilib>:"Add State(s) to Queue__jki_lib_state_machine.vi"("State(s) in (\"\")"=w412) -> ("States Out"=w411:string)  [unwired: 14 in]
      }
    }
  }
